vi "AO imaging_WF_20191030.vi"() -> ()   [LabVIEW 2018]
uses:
  Casao LabVIEW SDK 1.0.5/Haso/Data Haso/Wavefront parameters.ctl
  Casao LabVIEW SDK 1.0.5/Casao/Casao/Loop prefs.ctl
  Casao LabVIEW SDK 1.0.5/Haso/Data Haso/DataHaso.ctl
  <vilib>/Utility/file.llb/Read From Spreadsheet File (DBL).vi
  <vilib>/Utility/file.llb/Write To Spreadsheet File (DBL).vi
panel:
  in  "Stage Port":refnum<visa-resource-name>="COM5"
  in  "EMCCD fire port":tag="/Dev1/PFI0"
  in  "EMCCD trigger port":tag="Dev1/port0/line0"
  in  "Laser 2P shutter port":tag="Dev1/port0/line1"
  in  "Flip Mirror Port":tag="Dev1/ao5"
  in  "Laser 488 shutter port":tag="Dev1/port0/line3"
  out "error out 4":errorcluster
  out "error out 3":errorcluster
  out "error out 2":errorcluster
  out "error out":errorcluster
  out "output path":path
  out "Model Coefficients (µm) after":sgl[](array[numeric])
  out "Model Coefficients (µm) before":sgl[](array[numeric])
  in  "stop":bool
  out "Slice now":dbl
  in  "Iteration #":u16(ring)=1 items=["1"=1, "2"=2, "3"=3, "4"=4, "5"=5]
  in  "AoExp Time":dbl(ring)=0.5 items=["0.2s"=0.2, "0.5s"=0.5, "1.0s"=1.0, "1.5s"=1.5]
  out "after correction":T1
  in  "Filter y tilt":bool=TRUE
  in  "Filter x tilt":bool=TRUE
  in  "Curvature filter":bool=TRUE
  out "PV":dbl
  out "RMS":dbl
  in  "Matrix path":path=path "D:/Data/CM_20191031.aomc"
  in  "Offset path":path=path "D:/Data/system_aberration_20191029.dat"
  out "Camera image":u32[][](graph)
  out "RMS":dbl
  out "PV":dbl
  out "before correction":T1
  in  "Curvature filter":bool=TRUE
  in  "Filter y tilt":bool=TRUE
  in  "Filter x tilt":bool=TRUE
  out "after correction":dbl[][](graph) caption="Wavefront"
  out "before correction":dbl[][](graph) caption="Wavefront"
  in  "ImExp Time (s)":dbl(ring)=0.5 items=["0.2"=0.2, "0.5"=0.5, "1.0"=1.0, "4.0"=4.0, "8.0"=8.0]
  in  "Step size(um)":dbl
  in  "Slices #":dbl=2.0
  in  "Average Frame #":dbl=1.0
  in  "Correction":bool
  # "OFF"
  # "ON"
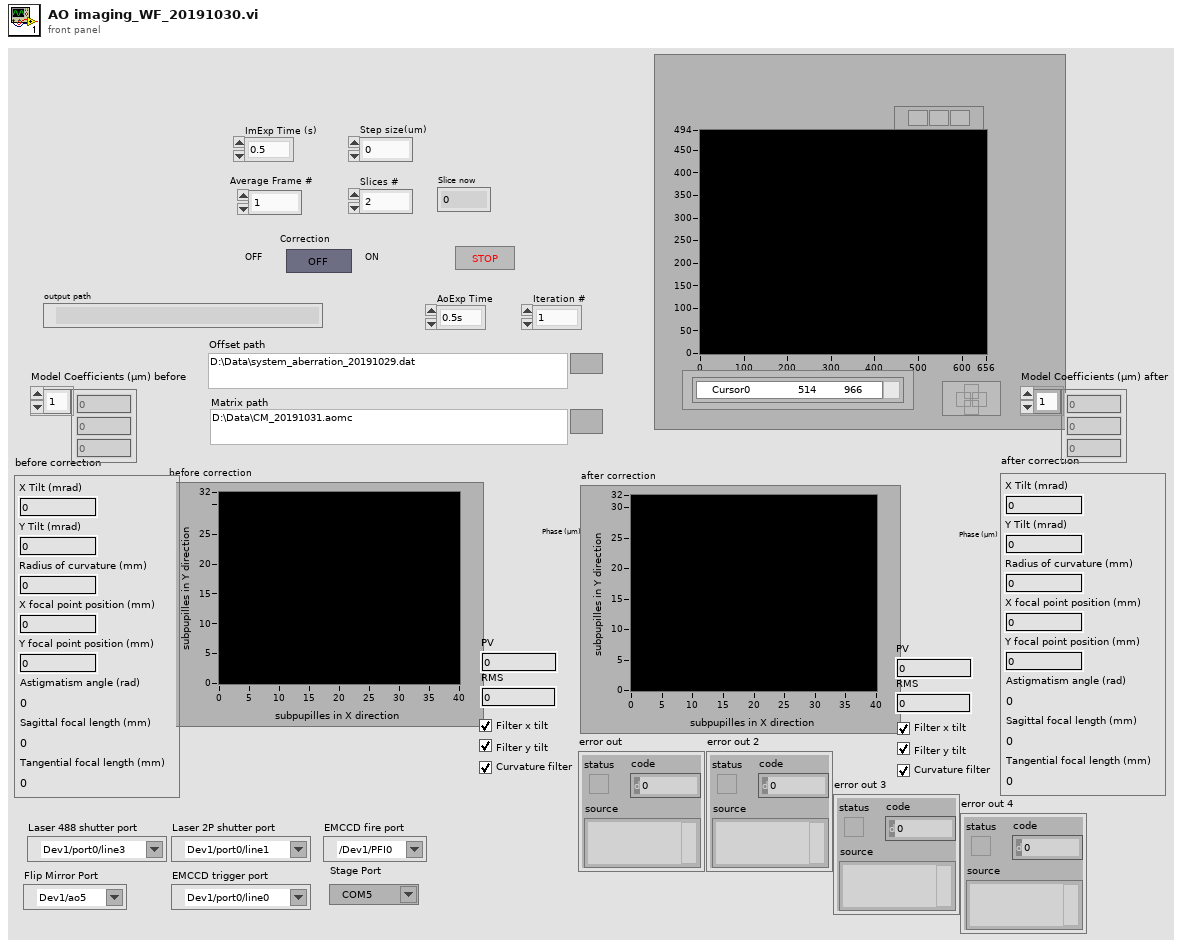
[diagram p1: front panel]
types:
  T1 = typedef "Wavefront parameters.ctl" = cluster{"X Tilt (mrad)":sgl, "Y Tilt (mrad)":sgl, "Radius of curvature (mm)":sgl, "X focal point position (mm)":sgl, "Y focal point position (mm)":sgl, "Astigmatism angle (rad)":sgl, "Sagittal focal length (mm)":sgl, "Tangential focal length (mm)":sgl}
  T2 = typedef "Loop prefs.ctl" = cluster{"Filter tilt on measurement (closed loop)":bool, "Correction gain (closed loop)":sgl, "Limit of subapertures off in CGP (%)":sgl, "Limit of saturated actuators (%)":sgl}
  T3 = cluster{"Filtre tilt X":bool, "Filtre tilt Y":bool, "Filtre courbure":bool}
  T4 = typedef "DataHaso.ctl" = i32
  T5 = cluster{"Measurement":T4, "Target":T4, "Manual target":T4}
  T6 = cluster{"Target for tilt":T4, "Target for focus":T4, "Target for all other aberrations":T4}
  T7 = typedef "Camera.ctl" = i32
  T8 = typedef "PhaseModul.ctl" = i32
  T9 = typedef "Haso.ctl" = i32
  T10 = typedef "Casao.ctl" = i32
  T11 = typedef "Image Compat.ctl" = cluster{"Signed/unsigned":bool, "Number of bits":T12, "Internal object id":i32, "Internal data id":i32}
  T12 = typedef "Data alignment enum.ctl" = enum16{"8", "16", "32"}
  T13 = typedef "Reconstruction prefs.ctl" = cluster{"Reconstruction type":enum16{"Modal", "Zonal"}, "Polynomial type":enum16{"Zernike", "Legendre"}, "Modal reconstruction prefs":T14, "Zonal reconstruction prefs":T17}
  T14 = typedef "Modal reconstruction prefs.ctl" = cluster{"Number of coefficients":u32, "Filtered coefficients":u32[], "RMS Zernike normalization":bool, "Matrix inversion method":u16, "Add zonal residual to modal fit ":bool, "Detection prefs":T15}
  T15 = typedef "PupilDetectionPrefs.ctl" = cluster{"Automatic pupil detection":bool, "Central occultation pupil":bool, "Semi-automatic pupil detection (find radius)":bool, "Semi-automatic pupil detection (find center)":bool, "Automatic pupil detection mode":enum16{"Contained", "Containing"}, "Start coordinates":cluster{"Pupil center (Zernike)":T16, "Pupil radius (Zernike)":sgl, "Pupil center (Legendre)":T16, "Pupil halfsize (Legendre)":T16}}
  T16 = typedef "Point2Df.ctl" = cluster{"X":sgl, "Y":sgl}
  T17 = typedef "Zonal reconstruction prefs.ctl" = cluster{"Number of weak iterations":u16, "Number of max iterations":u32, "Residual limit":sgl}
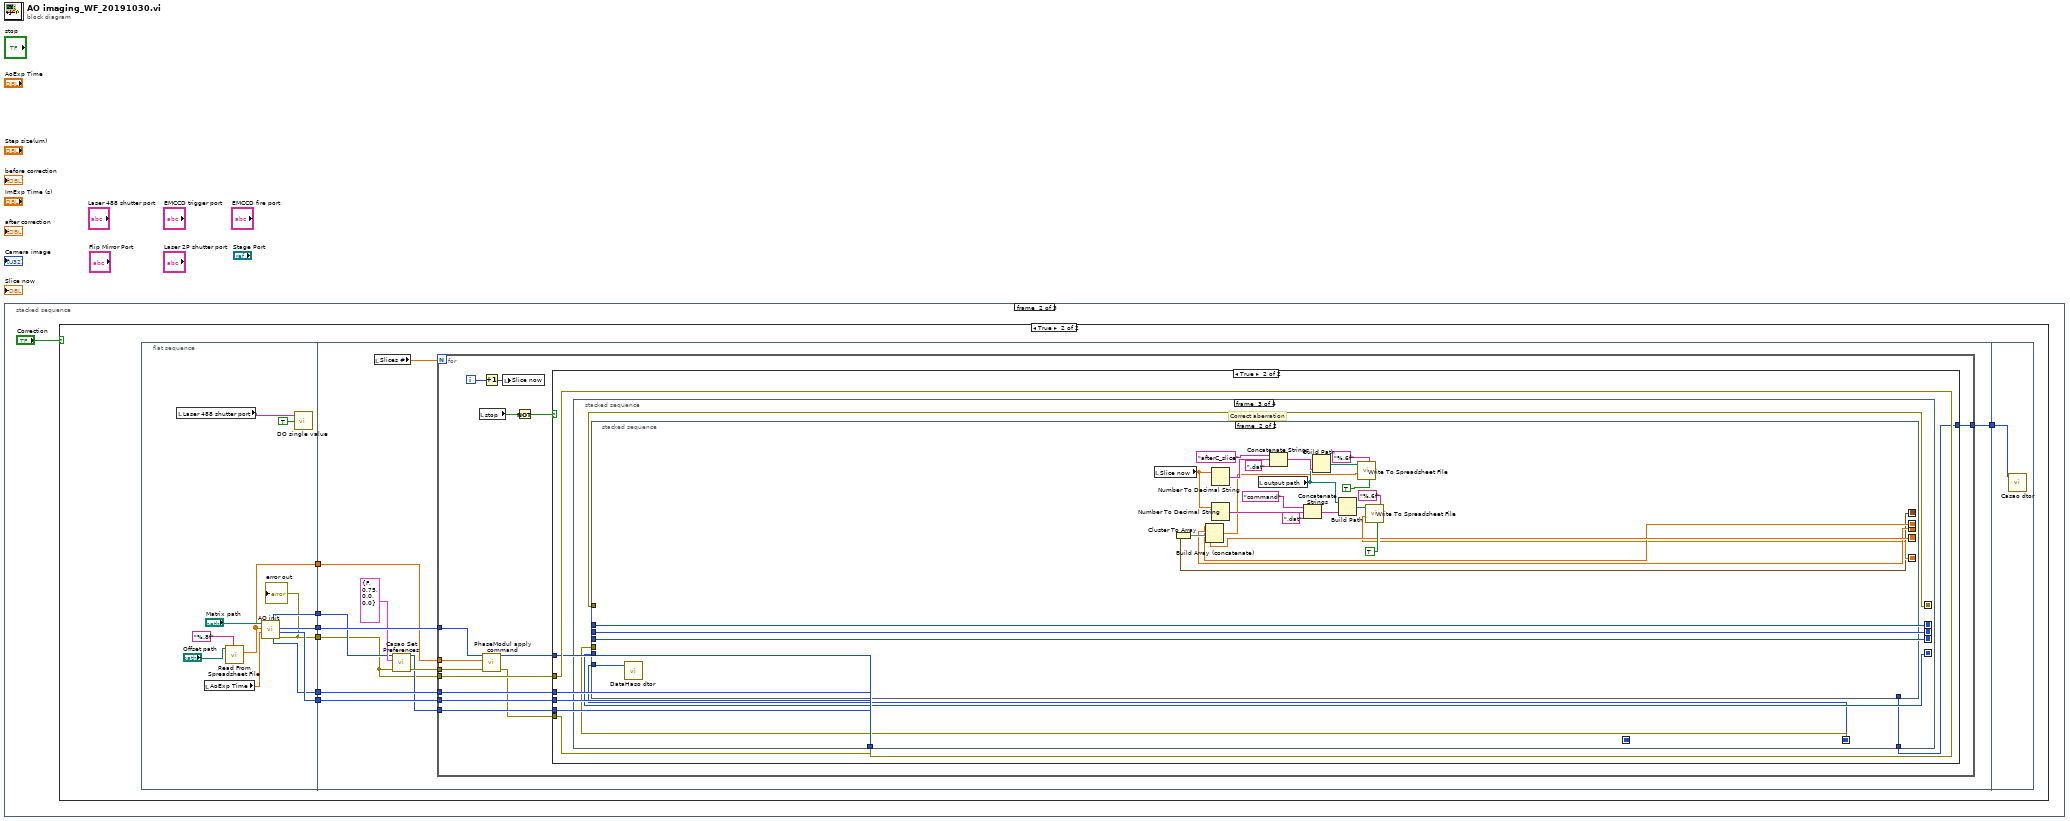
[diagram p0: block diagram]
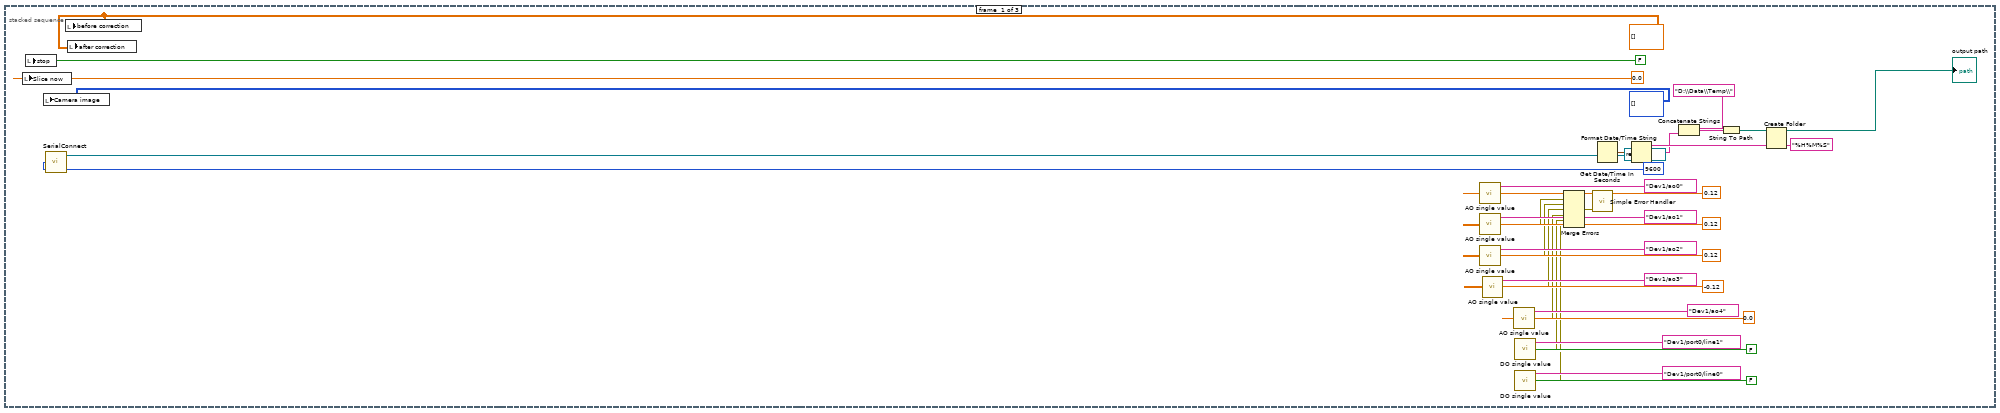
[diagram p2: hidden frame]
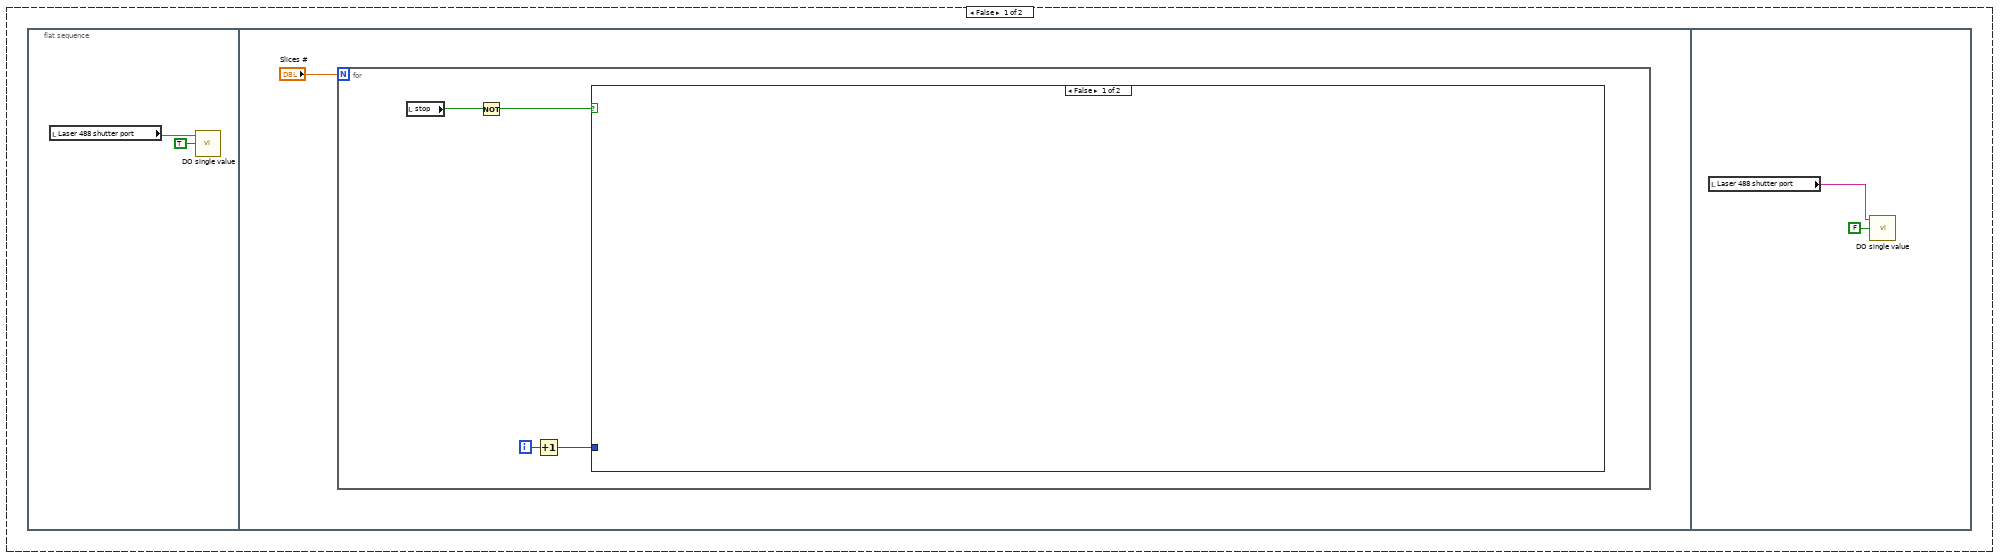
[diagram p3: hidden frame]
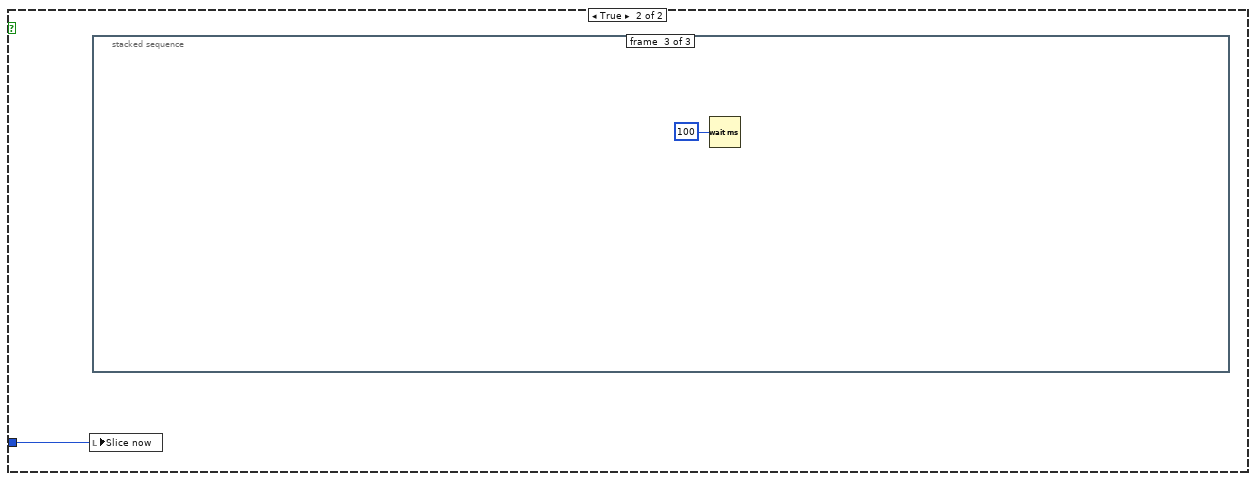
[diagram p4: hidden frame]
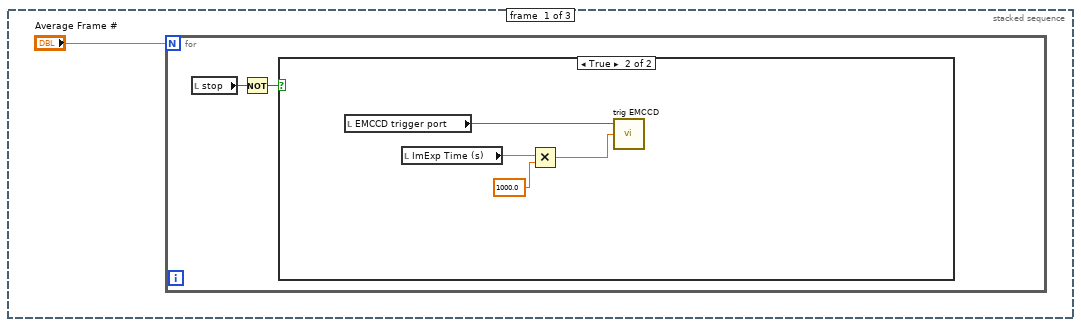
[diagram p5: hidden frame]
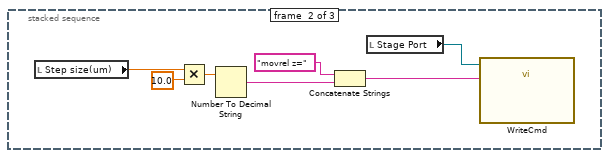
[diagram p7: hidden frame]
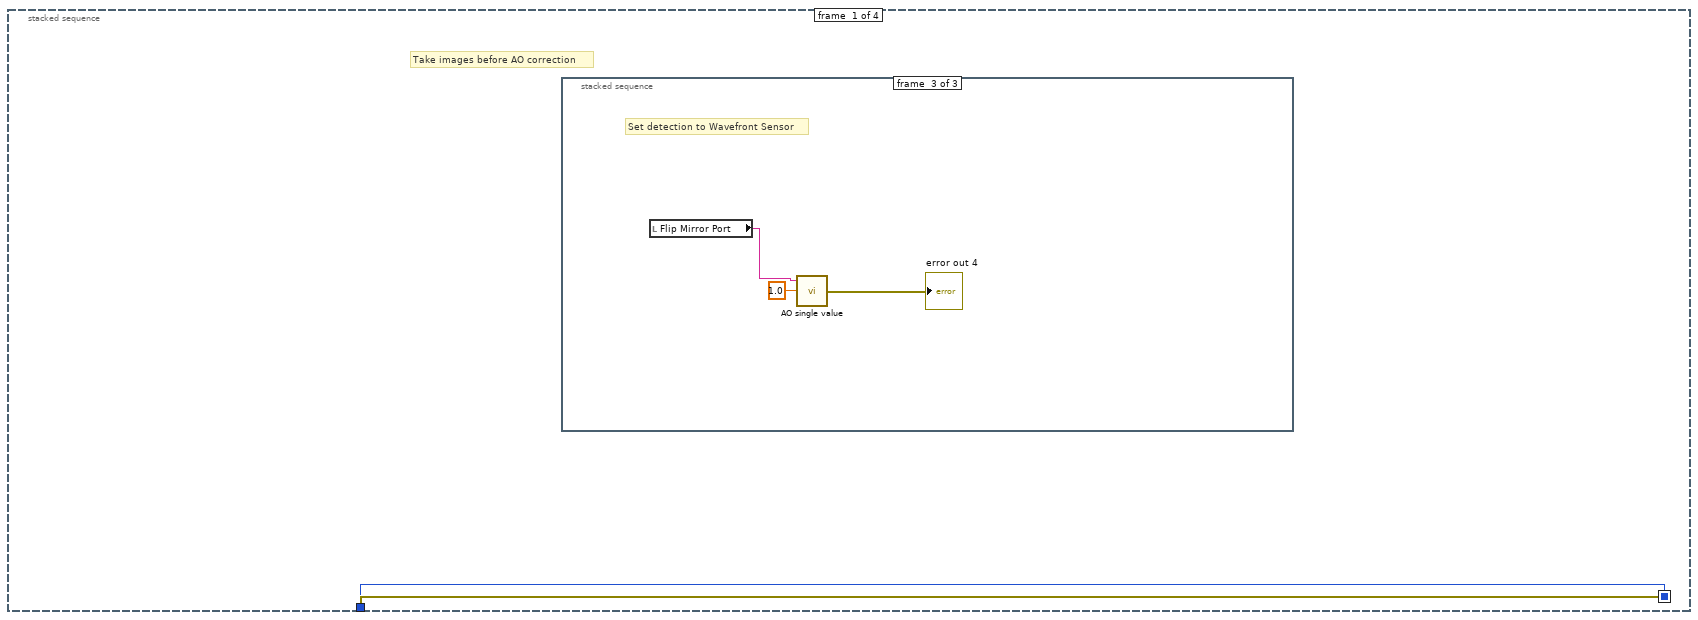
[diagram p9: hidden frame]
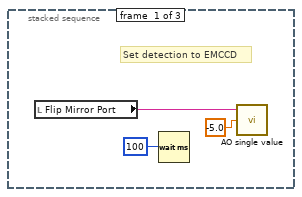
[diagram p10: hidden frame]
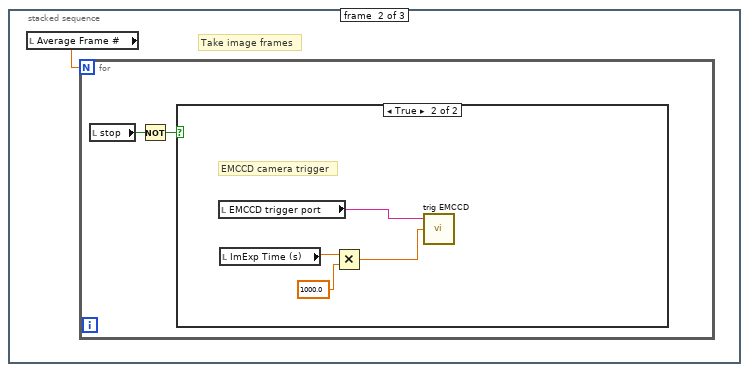
[diagram p11: hidden frame]
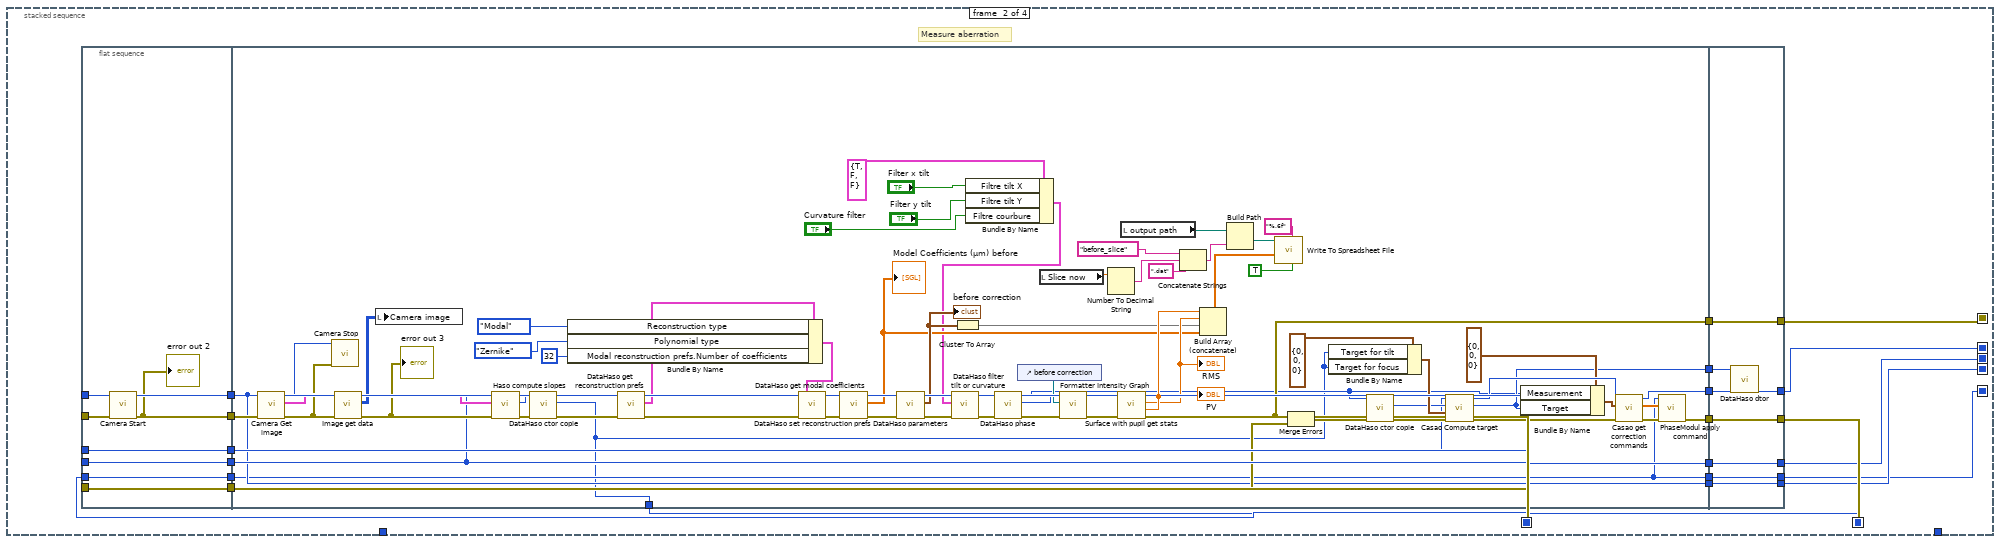
[diagram p13: hidden frame]
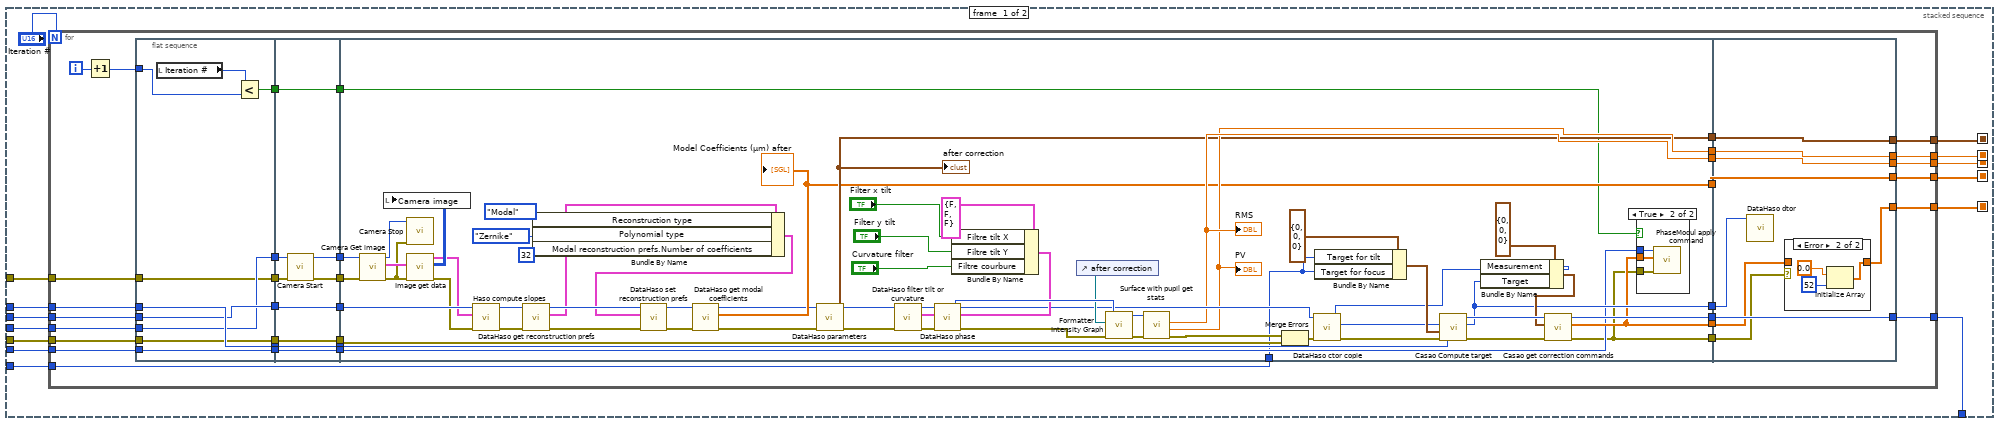
[diagram p14: hidden frame]
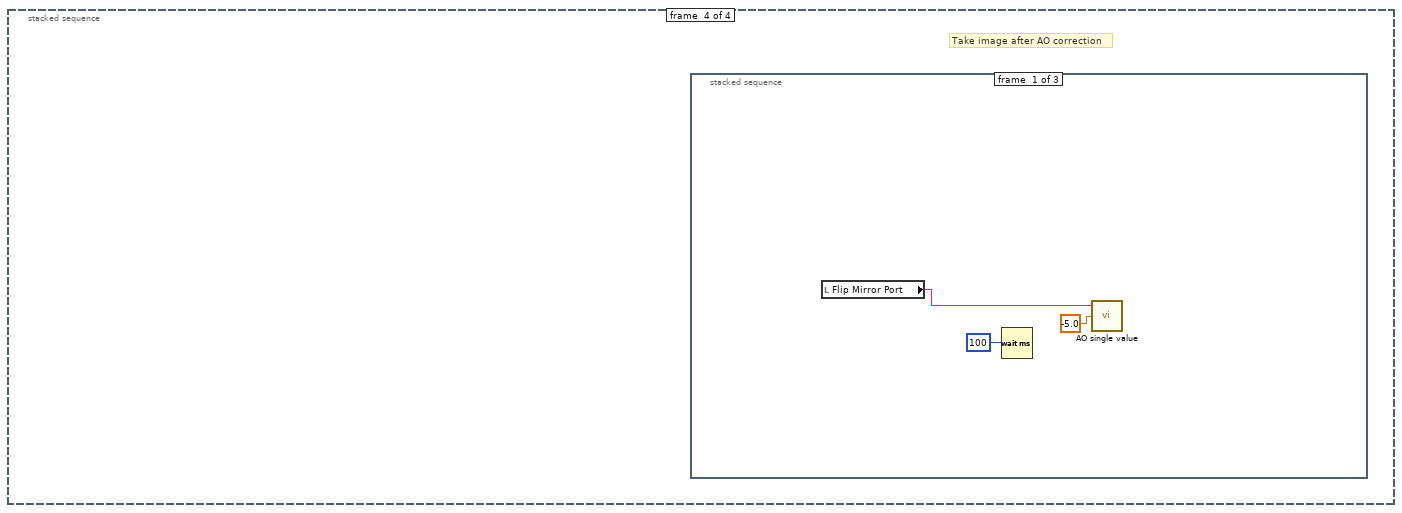
[diagram p17: hidden frame]
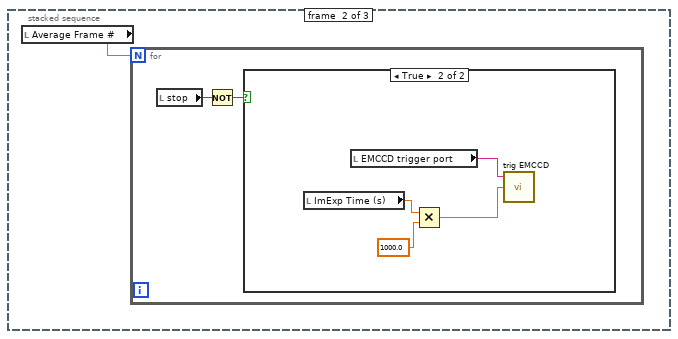
[diagram p18: hidden frame]
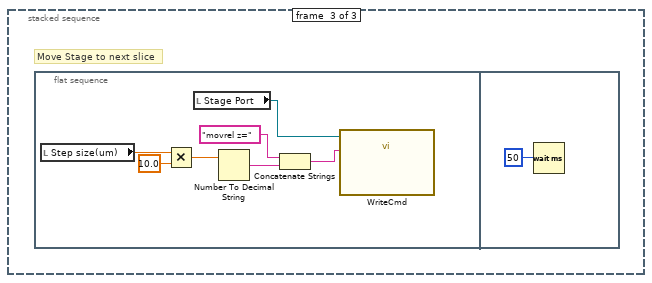
[diagram p20: hidden frame]
diagram:
  n1 = stacked-sequence {
    frame #0 {
      w34 = dbl[][] [] ("before correction")
      n2 = local write "Slice now"(0.0 ("Slice now")) -> ()
      n3 = local write "stop"(FALSE ("stop")) -> ()
      n4 = local write "Camera image"(u32[][] [] ("Camera image")) -> ()
      n5 = call "SerialConnect.vi"("baud rate (9600)"=u32 9600, "VISA resource name"=refnum<visa-resource-name> "COM1") -> ()  [unwired: 1 in, 3 out]
      n6 = local write "before correction"(w34) -> ()
      n7 = local write "after correction"(w34) -> ()
      n8 = call "AO single value.vi"("data"=0.12, "physical channels"=tag "Dev1/ao0") -> ("error out"=w17:errorcluster)  [unwired: 1 in]
      n9 = call "AO single value.vi"("data"=0.12, "physical channels"=tag "Dev1/ao1") -> ("error out"=w16:errorcluster)  [unwired: 1 in]
      n10 = call "AO single value.vi"("data"=0.12, "physical channels"=tag "Dev1/ao2") -> ("error out"=w15:errorcluster)  [unwired: 1 in]
      n11 = call "AO single value.vi"("data"=-0.12, "physical channels"=tag "Dev1/ao3") -> ("error out"=w14:errorcluster)  [unwired: 1 in]
      n12 = call "AO single value.vi"("data"=0.0, "physical channels"=tag "Dev1/ao4") -> ("error out"=w13:errorcluster)  [unwired: 1 in]
      n13 = call "DO single value.vi"("data"=FALSE, "lines"=tag "Dev1/port0/line1") -> ("error out"=w12:errorcluster)  [unwired: 1 in]
      n14 = call "DO single value.vi"("data"=FALSE, "lines"=tag "Dev1/port0/line0") -> ("error out"=w10:errorcluster)  [unwired: 1 in]
      n15 = Merge Errors(w17, w16, w15, w14, w13, w12, w10) -> (w11:errorcluster)
      n16 = call <vilib>:"Simple Error Handler.vi"("error in (no error)"=w11) -> ()  [unwired: 4 in, 5 out]
      n17 = Get Date/Time In Seconds() -> (seconds since 1Jan1904=w7:timestamp)
      n18 = Format Date/Time String(time format string (%c)="%H%M%S", seconds (now)=w7) -> (date/time string=w4:string)  [unwired: 1 in]
      n19 = Concatenate Strings("D:\\Data\\Temp\\" ("string"), w4) -> (w3:string)
      n20 = String To Path(string=w3) -> (path=w2:path)
      n21 = Create Folder(path (use dialog)=w2) -> (created path=→"output path":path)  [unwired: 2 in, 2 out]
    }
    frame #1 {
      n22 = case shown="True" "Correction" {
        frame False {
          n23 = flat-sequence {
            frame #0 {
              n24 = local read "Laser 488 shutter port"() -> (w37:tag)
              n25 = call "DO single value.vi"("data"=TRUE, "lines"=w37) -> ()  [unwired: 1 in, 1 out]
            }
            frame #1 {
              n26 = for {
                N: "Slices #" -> [_]
                i -> [w43]
                n27 = local read "stop"() -> (w41:bool)
                n28 = Not(x=w41) -> (.not. x?=w40:bool)
                n29 = Increment(x=w43) -> (x+1=w42:i32)
                n30 = case shown="False" w40 {
                  tunnel: w42 -> [_ w44]
                  frame False {
                  }
                  frame True {
                    n31 = local write "Slice now"(w44) -> ()
                    n32 = stacked-sequence {
                      frame #0 {
                        n33 = for {
                          N: "Average Frame #" -> [_]
                          n34 = local read "stop"() -> (w46:bool)
                          n35 = Not(x=w46) -> (.not. x?=w47:bool)
                          n36 = case shown="True" w47 {
                            frame False {
                            }
                            frame True {
                              n37 = local read "EMCCD trigger port"() -> (w48:tag)
                              n38 = local read "ImExp Time (s)"() -> (w49:dbl)
                              n39 = Multiply(x=w49, y=1000.0) -> (x*y=w50:dbl)
                              n40 = call "trig EMCCD.vi"("exp time (ms)"=w50, "lines"=w48) -> ()  [unwired: 1 in, 1 out]
                            }
                          }
                        }
                      }
                      frame #1 {
                        n41 = local read "Step size(um)"() -> (w53:dbl)
                        n42 = Multiply(x=w53, y=10.0) -> (x*y=w54:dbl)
                        n43 = Number To Decimal String(number=w54) -> (decimal integer string=w57:string)  [unwired: 1 in]
                        n44 = Concatenate Strings("movrel z=", w57) -> (w56:string)
                        n45 = local read "Stage Port"() -> (w52:refnum<visa-resource-name>)
                        n46 = call "WriteCmd.vi"("Command"=w56, "VISA resource name"=w52) -> ()  [unwired: 1 in, 1 out]
                      }
                      frame #2 {
                        n47 = Wait (ms)(milliseconds to wait=u32 100) -> ()  [unwired: 1 out]
                      }
                    }
                  }
                }
              }
            }
            frame #2 {
              n48 = local read "Laser 488 shutter port"() -> (w60:tag)
              n49 = call "DO single value.vi"("data"=FALSE, "lines"=w60) -> ()  [unwired: 1 in, 1 out]
            }
          }
        }
        frame True {
          n50 = flat-sequence {
            tunnel: [w75] -> w68
            tunnel: [w74] -> w67
            tunnel: [w70] -> w66
            tunnel: [w73] -> w65
            tunnel: [w72] -> w63
            tunnel: [w71] -> w62
            tunnel: w68 -> [w90]
            tunnel: w67 -> [w89]
            tunnel: w66 -> [w81]
            tunnel: w65 -> [w84]
            tunnel: [w88] -> w64
            tunnel: w63 -> [w87]
            tunnel: w62 -> [w82]
            tunnel: w64 -> [w443]
            frame #0 {
              n51 = local read "Laser 488 shutter port"() -> (w69:tag)
              n52 = local read "AoExp Time"() -> (w76:dbl)
              n53 = call-poly <vilib>:"Read From Spreadsheet File.vi"("format (%.3f)"="%.8f", "file path (dialog if empty)"="Offset path") -> ("first row"=w71:dbl[])  [unwired: 5 in, 4 out]
              n54 = call "AO init.vi"("Exposure duration specified (s)"=w76, "Commands in"=w71, "Matrix path"="Matrix path") -> ("error out"=w70:errorcluster, "Camera"=w75:T7, "Mirror"=w72:T8, "Haso"=w74:T9, "Casao"=w73:T10)  [unwired: 3 in, 1 out]
              "error out" <- w70
              n55 = call "DO single value.vi"("data"=TRUE, "lines"=w69) -> ()  [unwired: 1 in, 1 out]
            }
            frame #1 {
              n56 = local read "Slices #"() -> (w91:dbl)
              n57 = call "Casao Set Preferences.vi"("error in (no error)"=w81, "Loop preferences"=T2 {"Filter tilt on measurement (closed loop)"=FALSE, "Correction gain (closed loop)"=0.75, "Limit of subapertures off in CGP (%)"=0.0, "Limit of saturated actuators (%)"=0.0}, "Casao"=w84) -> ("error out"=w85:errorcluster, "Casao (dup)"=w83:T10)  [unwired: 3 in]
              n58 = for {
                N: w91 -> [_]
                tunnel: w81 -> [w105]
                tunnel: w90 -> [w104]
                tunnel: w89 -> [w103]
                tunnel: w85 -> [w93]
                tunnel: [w102] -> w88
                tunnel: w87 -> [w95]
                tunnel: w83 -> [w101]
                tunnel: w82 -> [w96]
                i -> [w97]
                n59 = local read "stop"() -> (w99:bool)
                n60 = Increment(x=w97) -> (x+1=w100:i32)
                n61 = call "PhaseModul apply command.vi"("error in (no error)"=w93, "Commands in"=w96, "Mirror"=w95) -> ("error out"=w92:errorcluster, "Mirror (dup)"=w94:T8)  [unwired: 2 in, 1 out]
                n62 = local write "Slice now"(w100) -> ()
                n63 = Not(x=w99) -> (.not. x?=w98:bool)
                n64 = case shown="True" w98 {
                  tunnel: w105 -> [_ w113]
                  tunnel: w104 -> [_ w112]
                  tunnel: w103 -> [_ w111]
                  tunnel: w92 -> [_ w110]
                  tunnel: [w106 w107] -> w102
                  tunnel: w94 -> [_ w109]
                  tunnel: w101 -> [w106 w108]
                  frame False {
                  }
                  frame True {
                    n65 = stacked-sequence {
                      seq-local: [w119 _ _ _] -> [_ w158 _ _]
                      seq-local: [w118 _ _ _] -> [_ w157 _ _]
                      seq-local: [w117 _ _ _] -> [_ w156 _ _]
                      seq-local: [w116 _ _ _] -> [_ w154 _ _]
                      seq-local: [w115 _ _ _] -> [_ w142 _ _]
                      seq-local: [w114 _ _ _] -> [_ w155 _ _]
                      seq-local: [_ w153 _ _] -> [_ _ w254 _]
                      seq-local: [_ w152 _ _] -> [_ _ w253 _]
                      seq-local: [_ w148 _ _] -> [_ _ w252 _]
                      seq-local: [_ w146 _ _] -> [_ _ w251 _]
                      seq-local: [_ w144 _ _] -> [_ _ w250 _]
                      seq-local: [_ w141 _ _] -> [_ _ w249 _]
                      seq-local: [_ w139 _ _] -> [_ _ w248 _]
                      tunnel: w113 -> [w119 _ _ _]
                      tunnel: w112 -> [w118 _ _ _]
                      tunnel: w111 -> [w117 _ _ _]
                      tunnel: w110 -> [w116 _ _ _]
                      tunnel: w109 -> [w115 _ _ _]
                      tunnel: w108 -> [w114 _ _ _]
                      tunnel: [_ _ w247 _] -> w107
                      frame #0 {
                        # "Take images before AO correction"
                        n66 = stacked-sequence {
                          frame #0 {
                            # "Set detection to EMCCD"
                            n67 = local read "Flip Mirror Port"() -> (w120:tag)
                            n68 = Wait (ms)(milliseconds to wait=u32 100) -> ()  [unwired: 1 out]
                            n69 = call "AO single value.vi"("data"=-5.0, "physical channels"=w120) -> ()  [unwired: 1 in, 1 out]
                          }
                          frame #1 {
                            # "Take image frames"
                            n70 = local read "Average Frame #"() -> (w123:dbl)
                            n71 = for {
                              N: w123 -> [_]
                              n72 = local read "stop"() -> (w124:bool)
                              n73 = Not(x=w124) -> (.not. x?=w125:bool)
                              n74 = case shown="True" w125 {
                                frame False {
                                }
                                frame True {
                                # "EMCCD camera trigger"
                                n75 = local read "EMCCD trigger port"() -> (w129:tag)
                                n76 = local read "ImExp Time (s)"() -> (w128:dbl)
                                n77 = Multiply(x=w128, y=1000.0) -> (x*y=w126:dbl)
                                n78 = call "trig EMCCD.vi"("exp time (ms)"=w126, "lines"=w129) -> ()  [unwired: 1 in, 1 out]
                                }
                              }
                            }
                          }
                          frame #2 {
                            # "Set detection to Wavefront Sensor"
                            n79 = local read "Flip Mirror Port"() -> (w130:tag)
                            n80 = call "AO single value.vi"("data"=1.0, "physical channels"=w130) -> ("error out"=→"error out 4":errorcluster)  [unwired: 1 in]
                          }
                        }
                      }
                      frame #1 {
                        # "Measure aberration"
                        n81 = flat-sequence {
                          tunnel: [w159] -> w138
                          tunnel: [w164] -> w137
                          tunnel: [w160] -> w136
                          tunnel: [w163] -> w135
                          tunnel: [w162] -> w134
                          tunnel: [w161] -> w133
                          tunnel: w158 -> [w165]
                          tunnel: w157 -> [w166]
                          tunnel: w156 -> [w159]
                          tunnel: w155 -> [w163]
                          tunnel: w154 -> [w162]
                          tunnel: w142 -> [w161]
                          tunnel: w136 -> [w239]
                          tunnel: w137 -> [w204]
                          tunnel: w138 -> [w205]
                          tunnel: w135 -> [w227]
                          tunnel: w134 -> [w226]
                          tunnel: [w208] -> w151
                          tunnel: [w207] -> w150
                          tunnel: [w206] -> w149
                          tunnel: [w205] -> w147
                          tunnel: [w204] -> w145
                          tunnel: [w203] -> w143
                          tunnel: w133 -> [w202]
                          tunnel: [w202] -> w140
                          tunnel: [w176] -> w139
                          tunnel: [w245] -> w152
                          tunnel: [w246] -> w153
                          tunnel: w151 -> [w246]
                          tunnel: w150 -> [w245]
                          tunnel: w149 -> [w244]
                          tunnel: [w243] -> w148
                          tunnel: w147 -> [w243]
                          tunnel: [w242] -> w146
                          tunnel: w145 -> [w242]
                          tunnel: [w241] -> w144
                          tunnel: w143 -> [w241]
                          tunnel: [w240] -> w141
                          tunnel: w140 -> [w240]
                          frame #0 {
                            n82 = call "Camera Start.vi"("error in (no error)"=w165, "camera"=w166) -> ("error out"=w160:errorcluster, "camera (dup)"=w164:T7)  [unwired: 4 in]
                            "error out 2" <- w160
                          }
                          frame #1 {
                            n83 = call "Camera Get image.vi"("error in (no error)"=w239, "camera"=w204) -> ("error out"=w223:errorcluster, "Image"=w224:T11, "camera (dup)"=w225:T7)  [unwired: 3 in]
                            n84 = call "Camera Stop.vi"("error in (no error)"=w223, "camera"=w225) -> ()  [unwired: 4 in, 2 out]
                            n85 = call "Image get data.vi"("error in (no error)"=w223, "Image Compat"=w224) -> ("error out"=w169:errorcluster, "Array"=w222:u32[][], "Image Compat (dup)"=w214:T11)  [unwired: 3 in]
                            "error out 3" <- w169
                            n86 = local write "Camera image"(w222) -> ()
                            n87 = call "Haso compute slopes.vi"("error in (no error)"=w169, "Image Compat"=w214, "Haso"=w205) -> ("error out"=w174:errorcluster, "Data Haso"=w178:T4)  [unwired: 1 in, 2 out]
                            n88 = call "DataHaso ctor copie.vi"("error in (no error)"=w174, "DataHaso"=w178) -> ("error out"=w173:errorcluster, "new DataHaso"=w176:T4, "DataHaso (dup)"=w175:T4)  [unwired: 3 in]
                            n89 = call "DataHaso get reconstruction prefs.vi"("error in (no error)"=w173, "Data Haso"=w175) -> ("error out"=w189:errorcluster, "Reconstruction Preferences"=w185:T13, "Data Haso (dup)"=w188:T4)  [unwired: 3 in]
                            n90 = Bundle By Name(cluster=w185, "Reconstruction type"=enum16{"Modal", "Zonal"}."Modal", "Polynomial type"=enum16{"Zernike", "Legendre"}."Zernike", "Modal reconstruction prefs.Number of coefficients"=u32 32) -> (w184:T13)
                            n91 = call "DataHaso set reconstruction prefs.vi"("error in (no error)"=w189, "Reconstruction Preferences"=w184, "Data Haso"=w188) -> ("error out"=w186:errorcluster, "Data Haso (dup)"=w187:T4)  [unwired: 3 in]
                            n92 = call "DataHaso get modal coefficients.vi"("error in (no error)"=w186, "Data Haso"=w187) -> ("error out"=w179:errorcluster, "Coefficients (µm)"=w190:sgl[], "Data Haso (dup)"=w180:T4)  [unwired: 3 in]
                            "Model Coefficients (µm) before" <- w190
                            n93 = call "DataHaso parameters.vi"("error in (no error)"=w179, "Data Haso"=w180) -> ("error out"=w220:errorcluster, "Parameters"=w198:T1, "Data Haso (dup)"=w221:T4)  [unwired: 3 in]
                            "before correction" <- w198
                            n94 = Cluster To Array(cluster=w198) -> (array=w199:sgl[])
                            n95 = Bundle By Name(cluster=T3 {"Filtre tilt X"=TRUE, "Filtre tilt Y"=FALSE, "Filtre courbure"=FALSE} ("Filtre"), "Filtre tilt X"="Filter x tilt", "Filtre tilt Y"="Filter y tilt", "Filtre courbure"="Curvature filter") -> (w167:T3)
                            n96 = call "DataHaso filter tilt or curvature.vi"("error in (no error)"=w220, "Filter (default: all true)"=w167, "Data Haso"=w221) -> ("error out"=w218:errorcluster, "Data Haso (dup)"=w219:T4)  [unwired: 3 in]
                            n97 = call "DataHaso phase.vi"("error in (no error)"=w218, "Data Haso"=w219) -> ("error out"=w217:errorcluster, "Phase (µm)"=w168:i32, "Data Haso (dup)"=w177:T4)  [unwired: 3 in]
                            n98 = control-ref of="before correction"() -> (w209:refnum<vi>)
                            n99 = local read "Slice now"() -> (w192:dbl)
                            n100 = call "Formatter Intensity Graph.vi"("error in (no error)"=w217, "Intensity Graph"=w209, "Surface with pupil"=w168) -> ("error out"=w215:errorcluster, "Surface with pupil (dup)"=w216:i32)  [unwired: 2 in, 1 out]
                            n101 = Number To Decimal String(number=w192) -> (decimal integer string=w194:string)  [unwired: 1 in]
                            n102 = call "Surface with pupil get stats.vi"("error in (no error)"=w215, "Surface Avec Pupille"=w216) -> ("error out"=w203:errorcluster, "PV"=w201:sgl, "RMS"=w200:dbl)  [unwired: 2 in, 1 out]
                            "PV" <- w201
                            "RMS" <- w200
                            n103 = local read "output path"() -> (w172:path)
                            n104 = Concatenate Strings("before_slice", w194, ".dat") -> (w171:string)
                            n105 = Build Array (concatenate)(w201, w200, w199, w190) -> (w197:dbl[])
                            n106 = Build Path(base path=w172, name or relative path=w171) -> (appended path=w170:path)
                            n107 = call-poly <vilib>:"Write To Spreadsheet File.vi"("transpose? (no:F)"=TRUE, "format (%.3f)"="%.6f", "1D data"=w197, "file path (dialog if empty)"=w170) -> ()  [unwired: 4 in, 1 out]
                            n108 = Merge Errors(w203, w226) -> (w234:errorcluster)
                            n109 = Bundle By Name(cluster=T6 {"Target for tilt"=0, "Target for focus"=0, "Target for all other aberrations"=0} ("References"), "Target for tilt"=w176, "Target for focus"=w176) -> (w237:T6)
                            n110 = call "DataHaso ctor copie.vi"("error in (no error)"=w234, "DataHaso"=w177) -> ("error out"=w236:errorcluster, "new DataHaso"=w235:T4)  [unwired: 3 in, 1 out]
                            n111 = call "Casao Compute target.vi"("error in (no error)"=w236, "Targets"=w237, "DataHaso"=w235, "Casao"=w227) -> ("error out"=w232:errorcluster, "DataHaso (dup)"=w206:T4, "Casao (dup)"=w233:T10)  [unwired: 1 out]
                            n112 = Bundle By Name(cluster=T5 {"Measurement"=0, "Target"=0, "Manual target"=0} ("Slopes"), "Measurement"=w177, "Target"=w206) -> (w231:T5)
                            n113 = call "Casao get correction commands.vi"("Casao"=w233, "Slopes"=w231, "error in (no error)"=w232) -> ("Casao (dup)"=w208:T10, "Commands"=w228:sgl[], "error out"=w229:errorcluster)  [unwired: 2 in, 2 out]
                            n114 = call "PhaseModul apply command.vi"("error in (no error)"=w229, "Commands in"=w228, "Mirror"=w202) -> ("error out"=w207:errorcluster)  [unwired: 2 in, 2 out]
                          }
                          frame #2 {
                            n115 = call "DataHaso dtor.vi"("Data Haso"=w244) -> ()  [unwired: 6 in, 1 out]
                          }
                        }
                      }
                      frame #2 {
                        # "Correct aberration"
                        n116 = stacked-sequence {
                          seq-local: [w261 _] -> [_ w405]
                          seq-local: [w260 _] -> [_ w404]
                          seq-local: [w259 _] -> [_ w402]
                          seq-local: [w258 _] -> [_ w403]
                          seq-local: [w257 _] -> [_ w406]
                          tunnel: w254 -> [w268 _]
                          tunnel: w253 -> [w267 _]
                          tunnel: w252 -> [w265 _]
                          tunnel: w251 -> [w264 _]
                          tunnel: w250 -> [w263 _]
                          tunnel: w249 -> [w262 _]
                          tunnel: w248 -> [w256 w401]
                          tunnel: [w255 _] -> w247
                          frame #0 {
                            n117 = for {
                              N: "Iteration #" -> [_]
                              tunnel: w268 -> [w300]
                              tunnel: w267 -> [w299]
                              tunnel: w265 -> [w298]
                              tunnel: w264 -> [w297]
                              tunnel: w263 -> [w296]
                              tunnel: [w294] -> w255
                              tunnel: w262 -> [w291]
                              tunnel: [w290] -> w261
                              tunnel: [w288] -> w260
                              tunnel: [w286] -> w259
                              tunnel: [w284] -> w258
                              tunnel: [w281] -> w257
                              tunnel: w256 -> [w280]
                              i -> [w279]
                              n118 = Increment(x=w279) -> (x+1=w278:i32)
                              n119 = flat-sequence {
                                tunnel: [w310] -> w305
                                tunnel: [w311] -> w304
                                tunnel: [w312] -> w303
                                tunnel: [w314] -> w302
                                tunnel: [w313] -> w301
                                tunnel: w300 -> [w314]
                                tunnel: w299 -> [w313]
                                tunnel: w298 -> [w312]
                                tunnel: w297 -> [w311]
                                tunnel: w296 -> [w310]
                                tunnel: [w309] -> w292
                                tunnel: w291 -> [w309]
                                tunnel: w278 -> [w307]
                                tunnel: [w306] -> w277
                                tunnel: w305 -> [w321]
                                tunnel: w304 -> [w322]
                                tunnel: w303 -> [w323]
                                tunnel: [w323] -> w275
                                tunnel: [w320] -> w274
                                tunnel: [w319] -> w273
                                tunnel: [w318] -> w272
                                tunnel: w302 -> [w318]
                                tunnel: [w317] -> w271
                                tunnel: w301 -> [w317]
                                tunnel: [w316] -> w270
                                tunnel: w292 -> [w316]
                                tunnel: [w315] -> w269
                                tunnel: w277 -> [w315]
                                tunnel: w273 -> [w382]
                                tunnel: w274 -> [w383]
                                tunnel: w275 -> [w384]
                                tunnel: w272 -> [w371]
                                tunnel: w271 -> [w370]
                                tunnel: [w350] -> w295
                                tunnel: [w349] -> w293
                                tunnel: w270 -> [w329]
                                tunnel: [w345] -> w289
                                tunnel: [w344] -> w287
                                tunnel: [w343] -> w285
                                tunnel: [w342] -> w283
                                tunnel: [w331] -> w282
                                tunnel: w280 -> [w328]
                                tunnel: w269 -> [w325]
                                tunnel: [w324] -> w276
                                tunnel: w295 -> [w396]
                                tunnel: [w395] -> w294
                                tunnel: w293 -> [w395]
                                tunnel: [w394] -> w290
                                tunnel: w289 -> [w394]
                                tunnel: [w393] -> w288
                                tunnel: w287 -> [w393]
                                tunnel: [w392] -> w286
                                tunnel: w285 -> [w392]
                                tunnel: [w388] -> w284
                                tunnel: w283 -> [w389]
                                tunnel: w282 -> [w391]
                                tunnel: [w391] -> w281
                                tunnel: w276 -> [w390]
                                frame #0 {
                                n120 = local read "Iteration #"() -> (w308:u16)
                                n121 = Less?(x=w308, y=w307) -> (x < y?=w306:bool)
                                }
                                frame #1 {
                                n122 = call "Camera Start.vi"("error in (no error)"=w321, "camera"=w322) -> ("error out"=w319:errorcluster, "camera (dup)"=w320:T7)  [unwired: 4 in]
                                }
                                frame #2 {
                                n123 = call "Camera Get image.vi"("error in (no error)"=w382, "camera"=w383) -> ("error out"=w367:errorcluster, "Image"=w368:T11, "camera (dup)"=w369:T7)  [unwired: 3 in]
                                n124 = call "Camera Stop.vi"("error in (no error)"=w367, "camera"=w369) -> ()  [unwired: 4 in, 2 out]
                                n125 = call "Image get data.vi"("error in (no error)"=w367, "Image Compat"=w368) -> ("error out"=w357:errorcluster, "Array"=w366:u32[][], "Image Compat (dup)"=w356:T11)  [unwired: 3 in]
                                n126 = local write "Camera image"(w366) -> ()
                                n127 = call "Haso compute slopes.vi"("error in (no error)"=w357, "Image Compat"=w356, "Haso"=w384) -> ("error out"=w334:errorcluster, "Data Haso"=w333:T4)  [unwired: 1 in, 2 out]
                                n128 = call "DataHaso get reconstruction prefs.vi"("error in (no error)"=w334, "Data Haso"=w333) -> ("error out"=w340:errorcluster, "Reconstruction Preferences"=w339:T13, "Data Haso (dup)"=w341:T4)  [unwired: 3 in]
                                n129 = Bundle By Name(cluster=w339, "Reconstruction type"=enum16{"Modal", "Zonal"}."Modal", "Polynomial type"=enum16{"Zernike", "Legendre"}."Zernike", "Modal reconstruction prefs.Number of coefficients"=u32 32) -> (w338:T13)
                                n130 = call "DataHaso set reconstruction prefs.vi"("error in (no error)"=w340, "Reconstruction Preferences"=w338, "Data Haso"=w341) -> ("error out"=w326:errorcluster, "Data Haso (dup)"=w327:T4)  [unwired: 3 in]
                                n131 = call "DataHaso get modal coefficients.vi"("error in (no error)"=w326, "Data Haso"=w327) -> ("error out"=w332:errorcluster, "Coefficients (µm)"=w331:sgl[], "Data Haso (dup)"=w330:T4)  [unwired: 3 in]
                                "Model Coefficients (µm) after" <- w331
                                n132 = call "DataHaso parameters.vi"("error in (no error)"=w332, "Data Haso"=w330) -> ("error out"=w364:errorcluster, "Parameters"=w343:T1, "Data Haso (dup)"=w365:T4)  [unwired: 3 in]
                                "after correction" <- w343
                                n133 = Bundle By Name(cluster=T3 {"Filtre tilt X"=FALSE, "Filtre tilt Y"=FALSE, "Filtre courbure"=FALSE} ("Filtre"), "Filtre tilt X"="Filter x tilt", "Filtre tilt Y"="Filter y tilt", "Filtre courbure"="Curvature filter") -> (w354:T3)
                                n134 = call "DataHaso filter tilt or curvature.vi"("error in (no error)"=w364, "Filter (default: all true)"=w354, "Data Haso"=w365) -> ("error out"=w362:errorcluster, "Data Haso (dup)"=w363:T4)  [unwired: 3 in]
                                n135 = call "DataHaso phase.vi"("error in (no error)"=w362, "Data Haso"=w363) -> ("error out"=w360:errorcluster, "Phase (µm)"=w361:i32, "Data Haso (dup)"=w347:T4)  [unwired: 3 in]
                                n136 = control-ref of="after correction"() -> (w348:refnum<vi>)
                                n137 = call "Formatter Intensity Graph.vi"("error in (no error)"=w360, "Intensity Graph"=w348, "Surface with pupil"=w361) -> ("error out"=w358:errorcluster, "Surface with pupil (dup)"=w359:i32)  [unwired: 2 in, 1 out]
                                n138 = call "Surface with pupil get stats.vi"("error in (no error)"=w358, "Surface Avec Pupille"=w359) -> ("error out"=w377:errorcluster, "PV"=w344:sgl, "RMS"=w345:dbl)  [unwired: 2 in, 1 out]
                                "RMS" <- w345
                                "PV" <- w344
                                n139 = Merge Errors(w377, w370) -> (w376:errorcluster)
                                n140 = call "DataHaso ctor copie.vi"("error in (no error)"=w376, "DataHaso"=w347) -> ("error out"=w379:errorcluster, "new DataHaso"=w378:T4, "DataHaso (dup)"=w346:T4)  [unwired: 3 in]
                                n141 = Bundle By Name(cluster=T6 {"Target for tilt"=0, "Target for focus"=0, "Target for all other aberrations"=0} ("References"), "Target for tilt"=w328, "Target for focus"=w328) -> (w380:T6)
                                n142 = call "Casao Compute target.vi"("error in (no error)"=w379, "Targets"=w380, "DataHaso"=w378, "Casao"=w371) -> ("error out"=w374:errorcluster, "DataHaso (dup)"=w350:T4, "Casao (dup)"=w375:T10)  [unwired: 1 out]
                                n143 = Bundle By Name(cluster=T5 {"Measurement"=0, "Target"=0, "Manual target"=0} ("Slopes"), "Measurement"=w346, "Target"=w350) -> (w373:T5)
                                n144 = call "Casao get correction commands.vi"("Casao"=w375, "Slopes"=w373, "error in (no error)"=w374) -> ("Casao (dup)"=w349:T10, "Commands"=w342:sgl[], "error out"=w324:errorcluster)  [unwired: 2 in, 2 out]
                                n145 = case shown="True" w325 {
                                tunnel: w324 -> [_ w387]
                                tunnel: w342 -> [_ w386]
                                tunnel: w329 -> [_ w385]
                                frame False {
                                }
                                frame True {
                                n146 = call "PhaseModul apply command.vi"("error in (no error)"=w387, "Commands in"=w386, "Mirror"=w385) -> ()  [unwired: 2 in, 3 out]
                                }
                                }
                                }
                                frame #3 {
                                n147 = call "DataHaso dtor.vi"("Data Haso"=w396) -> ()  [unwired: 6 in, 1 out]
                                n148 = case shown="Error" w390 {
                                tunnel: w389 -> [w397 _]
                                tunnel: [w397 w398] -> w388
                                frame No Error {
                                }
                                frame Error {
                                n149 = Initialize Array(0.0 ("element"), 52 ("dimension size")) -> (w398:dbl[])
                                }
                                }
                                }
                              }
                            }
                          }
                          frame #1 {
                            n150 = call "DataHaso dtor.vi"("Data Haso"=w401) -> ()  [unwired: 6 in, 1 out]
                            n151 = local read "Slice now"() -> (w419:dbl)
                            n152 = Cluster To Array(cluster=w402) -> (array=w417:sgl[])
                            n153 = Build Array (concatenate)(w404, w405, w417, w406) -> (w415:dbl[])
                            n154 = Number To Decimal String(number=w419) -> (decimal integer string=w416:string)  [unwired: 1 in]
                            n155 = Number To Decimal String(number=w419) -> (decimal integer string=w418:string)  [unwired: 1 in]
                            n156 = local read "output path"() -> (w420:path)
                            n157 = Concatenate Strings("afterC_slice", w416, ".dat") -> (w421:string)
                            n158 = Concatenate Strings("command", w418, ".dat") -> (w423:string)
                            n159 = Build Path(base path=w420, name or relative path=w421) -> (appended path=w422:path)
                            n160 = Build Path(base path=w420, name or relative path=w423) -> (appended path=w424:path)
                            n161 = call-poly <vilib>:"Write To Spreadsheet File.vi"("transpose? (no:F)"=TRUE, "format (%.3f)"="%.6f", "1D data"=w415, "file path (dialog if empty)"=w422) -> ()  [unwired: 4 in, 1 out]
                            n162 = call-poly <vilib>:"Write To Spreadsheet File.vi"("transpose? (no:F)"=TRUE, "format (%.3f)"="%.6f", "1D data"=w403, "file path (dialog if empty)"=w424) -> ()  [unwired: 4 in, 1 out]
                          }
                        }
                      }
                      frame #3 {
                        # "Take image after AO correction"
                        n163 = stacked-sequence {
                          frame #0 {
                            n164 = local read "Flip Mirror Port"() -> (w425:tag)
                            n165 = Wait (ms)(milliseconds to wait=u32 100) -> ()  [unwired: 1 out]
                            n166 = call "AO single value.vi"("data"=-5.0, "physical channels"=w425) -> ()  [unwired: 1 in, 1 out]
                          }
                          frame #1 {
                            n167 = local read "Average Frame #"() -> (w428:dbl)
                            n168 = for {
                              N: w428 -> [_]
                              n169 = local read "stop"() -> (w429:bool)
                              n170 = Not(x=w429) -> (.not. x?=w430:bool)
                              n171 = case shown="True" w430 {
                                frame False {
                                }
                                frame True {
                                n172 = local read "ImExp Time (s)"() -> (w431:dbl)
                                n173 = local read "EMCCD trigger port"() -> (w432:tag)
                                n174 = Multiply(x=w431, y=1000.0) -> (x*y=w433:dbl)
                                n175 = call "trig EMCCD.vi"("exp time (ms)"=w433, "lines"=w432) -> ()  [unwired: 1 in, 1 out]
                                }
                              }
                            }
                          }
                          frame #2 {
                            # "Move Stage to next slice"
                            n176 = flat-sequence {
                              frame #0 {
                                n177 = local read "Step size(um)"() -> (w438:dbl)
                                n178 = Multiply(x=w438, y=10.0) -> (x*y=w439:dbl)
                                n179 = local read "Stage Port"() -> (w435:refnum<visa-resource-name>)
                                n180 = Number To Decimal String(number=w439) -> (decimal integer string=w441:string)  [unwired: 1 in]
                                n181 = Concatenate Strings("movrel z=", w441) -> (w440:string)
                                n182 = call "WriteCmd.vi"("Command"=w440, "VISA resource name"=w435) -> ()  [unwired: 1 in, 1 out]
                              }
                              frame #1 {
                                n183 = Wait (ms)(milliseconds to wait=u32 50) -> ()  [unwired: 1 out]
                              }
                            }
                          }
                        }
                      }
                    }
                  }
                }
              }
            }
            frame #2 {
              n184 = call "Casao dtor.vi"("Casao"=w443) -> ()  [unwired: 6 in, 1 out]
            }
          }
        }
      }
    }
    frame #2 {
      n185 = local read "Step size(um)"() -> (w451:dbl)
      n186 = local read "Slices #"() -> (w445:dbl)
      n187 = Multiply(x=w451, y=-10.0) -> (x*y=w452:dbl)
      n188 = Multiply(x=w452, y=w445) -> (x*y=w450:dbl)
      n189 = Number To Decimal String(number=w450) -> (decimal integer string=w447:string)  [unwired: 1 in]
      n190 = Concatenate Strings("movrel z=", w447) -> (w448:string)
      n191 = call "AO single value.vi"("data"=0.0, "physical channels"=tag "Dev1/ao4") -> ()  [unwired: 1 in, 1 out]
      n192 = call "DO single value.vi"("data"=FALSE, "lines"=tag "Dev1/port0/line1") -> ()  [unwired: 1 in, 1 out]
      n193 = call "DO single value.vi"("data"=FALSE, "lines"=tag "Dev1/port0/line0") -> ()  [unwired: 1 in, 1 out]
      n194 = local read "Stage Port"() -> (w444:refnum<visa-resource-name>)
      n195 = call "WriteCmd.vi"("Command"=w448, "VISA resource name"=w444) -> ()  [unwired: 1 in, 1 out]
    }
  }
